vi "DDOdom_Abs_Traj_Exec.vi"(11 "Init":bool) -> (0 "Odom Pose Eng":T1 {"ROTATION"."SIN" format="%13.4f"; "ROTATION"."COS" format="%13.4f"; "ROTATION"."VALUE" format="%13.4f"; "TRANSLATION"."Y" format="%14.3f"; "TRANSLATION"."X" format="%14.3f"}, 1 "AtReference":bool, 2 "Right Speed Target":dbl, 3 "Left Speed Target":dbl)   [LabVIEW 2019]
uses:
  <vilib>/Rock Robotics/WPI/ThirdParty/JAS_Junk/TrajLib/TypeDef/POSE2D.ctl
  <vilib>/Rock Robotics/WPI/ThirdParty/JAS_Junk/TrajLib/TypeDef/TRANSLATION2D.ctl
  <vilib>/Rock Robotics/WPI/ThirdParty/JAS_Junk/TrajLib/TypeDef/ROTATION2D.ctl
  <vilib>/Rock Robotics/WPI/ThirdParty/JAS_Junk/TrajLib/Conv_Meters_Feet.vi
  <vilib>/Rock Robotics/WPI/ThirdParty/JAS_Junk/TrajLib/Conv_Radians_Deg.vi
  <vilib>/Rock Robotics/WPI/ThirdParty/JAS_Junk/TrajLib/Trajectory_Library.lvlib
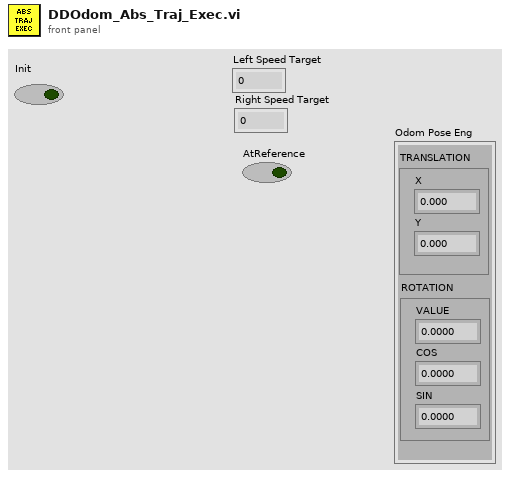
[diagram p1: front panel]
types:
  T1 = typedef "Trajectory_Library.lvlib/POSE2D.ctl" = cluster{"TRANSLATION":T2, "ROTATION":T3}
  T2 = typedef "Trajectory_Library.lvlib/TRANSLATION2D.ctl" = cluster{"X":dbl, "Y":dbl}
  T3 = typedef "Trajectory_Library.lvlib/ROTATION2D.ctl" = cluster{"VALUE":dbl, "COS":dbl, "SIN":dbl}
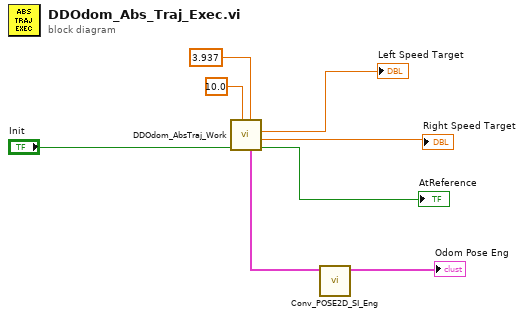
[diagram p0: block diagram]
diagram:
  n1 = call "DDOdom_AbsTraj_Work.vi"("Track Width FT"=3.937, "Max Speed\nFT/SEC"=10.0 ("Max Speed\nFT/SEC"), "Init"="Init") -> ("AtReference"=→"AtReference":bool, "Right Speed Target"=→"Right Speed Target":dbl, "Left Speed Target"=→"Left Speed Target":dbl, "Odometry Pose Meters"=w2:T1)  [unwired: 5 in]
  n2 = call <vilib>:"Conv_POSE2D_SI_Eng.vi"("Err Pose in SI"=w2) -> ("Err Pose out ENG"=→"Odom Pose Eng":T1)  [unwired: 10 in]
